vi "UI_Alarm_Settings_Sensor.vi"() -> ()   [LabVIEW 2014]
uses:
  <vilib>/addons/database/NI_Database_API.lvlib
  <vilib>/addons/database/Connection.llb/DB Tools Open Connec (String).vi
  <vilib>/addons/database/Connection.llb/Conn Execute.vi
  <vilib>/addons/database/Recordset.llb/Rec Destroy - Connection.vi
panel:
  in  "退出":bool
  in  "转速":u16(ring) items=["L0", "L1", "L2", "L3"]
  in  "径向位移":u16(ring) items=["L0", "L1", "L2", "L3"]
  in  "2X/2Y位移":u16(ring) items=["L0", "L1", "L2", "L3"]
  in  "主轴检测单元":string[][](table)
  in  "保存":bool
  in  "编辑":bool
  in  "轴向油缸力":u16(ring) items=["L0", "L1", "L2", "L3"]
  in  "径向油缸力":u16(ring) items=["L0", "L1", "L2", "L3"]
  in  "轴承外圈温度":u16(ring) items=["L0", "L1", "L2", "L3"]
  in  "声发射频率":u16(ring) items=["L0", "L1", "L2", "L3"]
  in  "声发射幅度":u16(ring) items=["L0", "L1", "L2", "L3"]
  in  "出油温度":u16(ring) items=["L0", "L1", "L2", "L3"]
  in  "摩擦力矩1":u16(ring) items=["L0", "L1", "L2", "L3"]
  in  "摩擦力矩2":u16(ring) items=["L0", "L1", "L2", "L3"]
  in  "外壳振动":u16(ring) items=["L0", "L1", "L2", "L3"]
  in  "陪试温度":u16(ring) items=["L0", "L1", "L2", "L3"]
  in  "加载单元":string[][](table)
  in  "陪试轴承润滑单元":string[][](table)
  in  "实验轴承单元":string[][](table)
  # "工作参数报警门限设置"
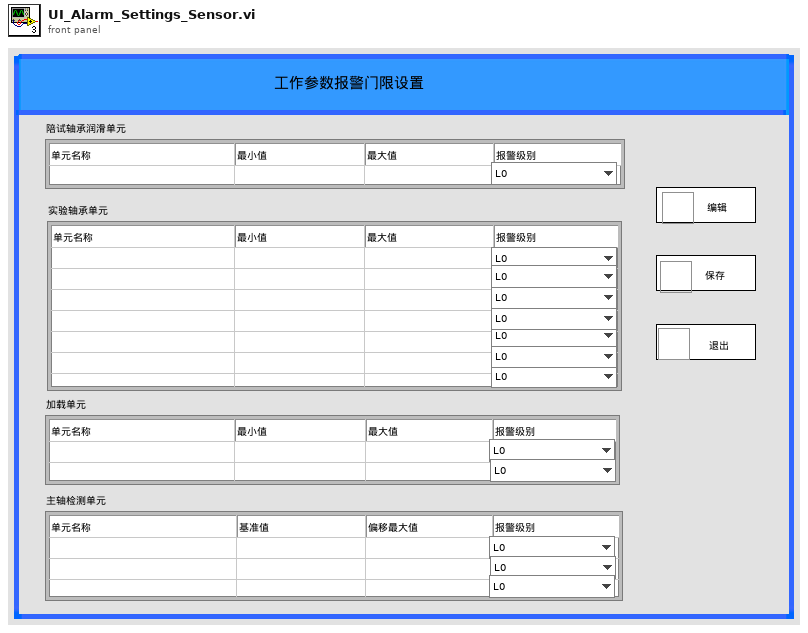
[diagram p1: front panel]
types:
  T1 = typedef "NI_Database_API.lvlib/Conn ObjectReference.ctl" = refnum<k1>
  T2 = typedef "NI_Database_API.lvlib/Rec ObjectReference.ctl" = refnum<k1>
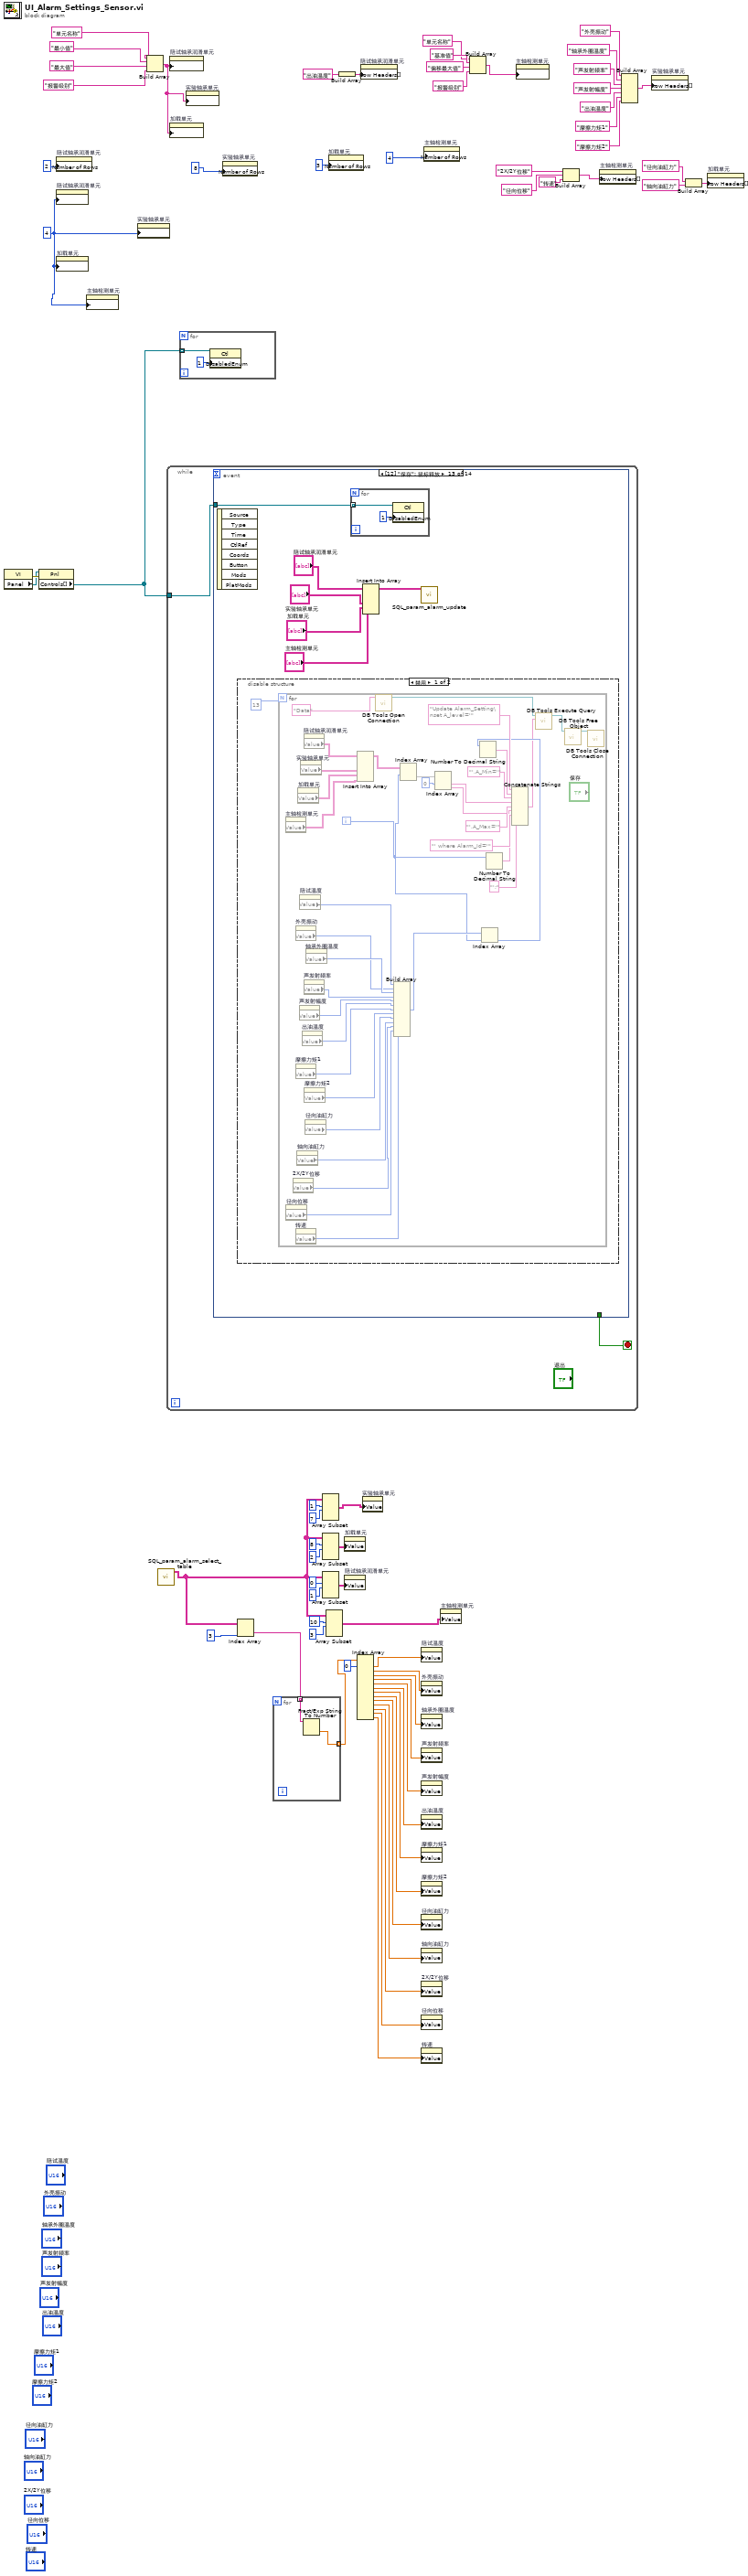
[diagram p0: block diagram]
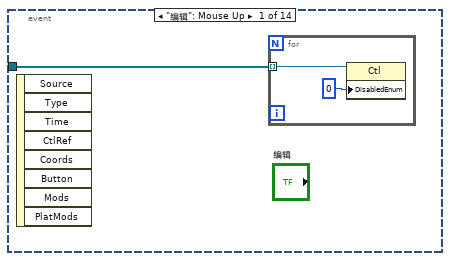
[diagram p2: hidden frame]
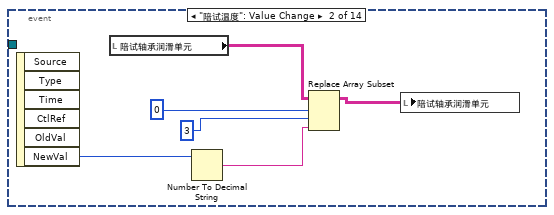
[diagram p3: hidden frame]
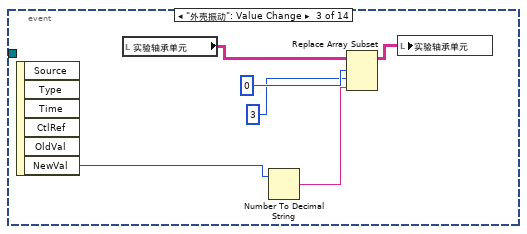
[diagram p4: hidden frame]
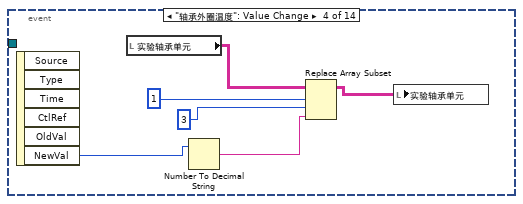
[diagram p5: hidden frame]
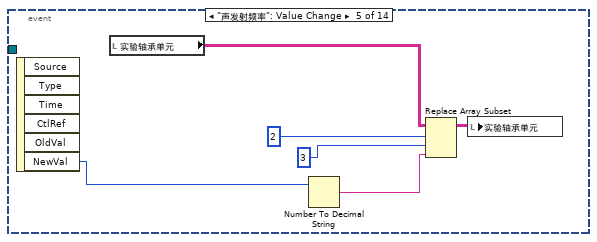
[diagram p6: hidden frame]
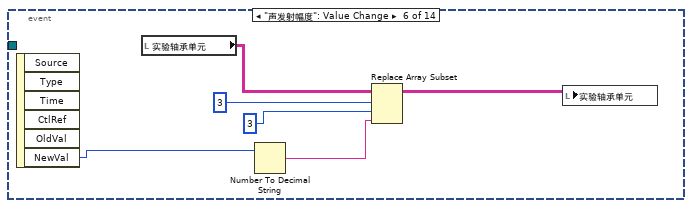
[diagram p7: hidden frame]
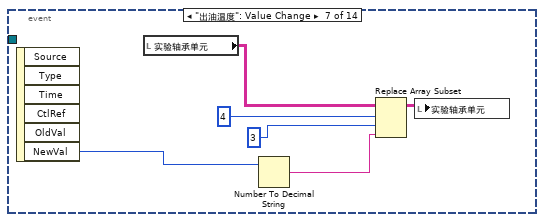
[diagram p8: hidden frame]
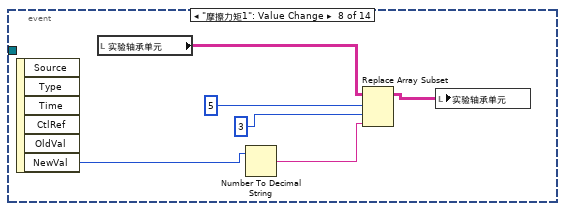
[diagram p9: hidden frame]
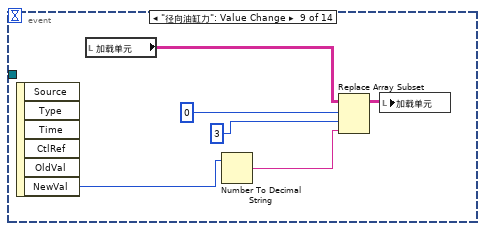
[diagram p10: hidden frame]
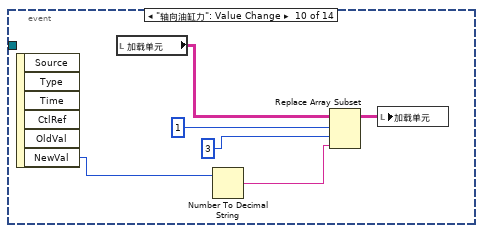
[diagram p11: hidden frame]
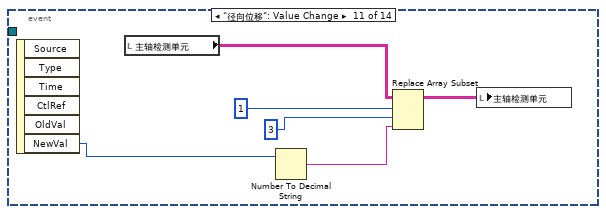
[diagram p12: hidden frame]
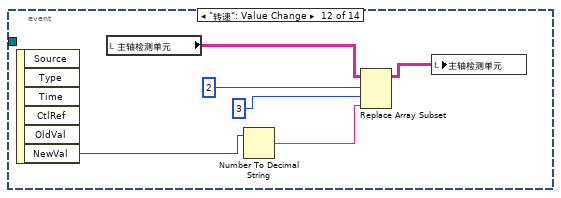
[diagram p13: hidden frame]
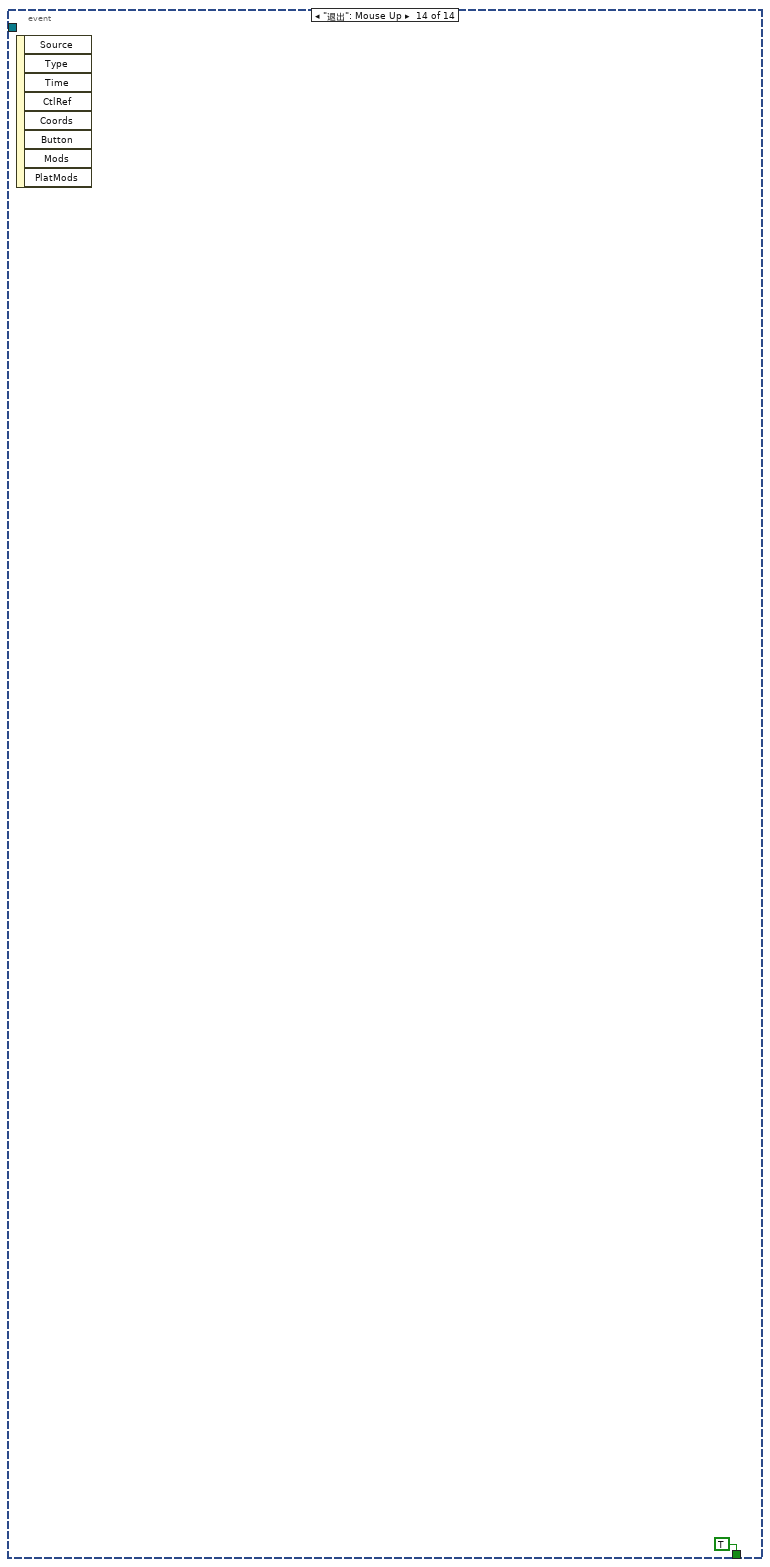
[diagram p15: hidden frame]
diagram:
  w34 = 4
  n1 = property class="VI"() -> (error out=w49:errorcluster, "Panel"=w48:refnum<vi>)  [unwired: 2 in, 1 out]
  n2 = property class="Pnl"(reference=w48, error in=w49) -> ("Controls[]"=w47:refnum<vi>[])  [unwired: 2 out]
  n3 = property on="陪试轴承润滑单元" class="Tbl (严格)"("Number of Rows"=2) -> ()  [unwired: 2 in, 2 out]
  n4 = property on="陪试轴承润滑单元" class="Tbl (严格)"("Number of Columns"=w34) -> ()  [unwired: 2 in, 2 out]
  n5 = property on="加载单元" class="Tbl (严格)"("Number of Columns"=w34) -> ()  [unwired: 2 in, 2 out]
  n6 = property on="主轴检测单元" class="Tbl (严格)"("Number of Columns"=w34) -> ()  [unwired: 2 in, 2 out]
  n7 = property on="实验轴承单元" class="Tbl (严格)"("Number of Columns"=w34) -> ()  [unwired: 2 in, 2 out]
  n8 = Build Array("单元名称", "最小值", "最大值", "报警级别") -> (w38:string[])
  n9 = call "SQL_param_alarm_select_table.vi"() -> ("表格控件"=w4:string[][])  [unwired: 10 in, 1 out]
  n10 = while {
    tunnel: w47 -> [w67]
    stop <- w66 stop-if-true
    n11 = event shown="[12] \"保存\": 鼠标释放" {
      selector: _ -> [_ _ _ _ _ _ _ _ _ _ _ _ _ _]
      dyn-events: _ -> [_ _ _ _ _ _ _ _ _ _ _ _ _ _]
      timeout: _ -> [_ _ _ _ _ _ _ _ _ _ _ _ _ _]
      tunnel: w67 -> [w68 _ _ _ _ _ _ _ _ _ _ _ w142 _]
      tunnel: [_ _ _ _ _ _ _ _ _ _ _ _ _ TRUE] -> w66
      event "编辑": Mouse Up {
        n12 = event-data() -> ()  [unwired: 1 in, 8 out]
        n13 = for {
          tunnel: w68 -> [w70] mode=indexing
          n14 = property class="Ctl"(reference=w70, "DisabledEnum"=0) -> ()  [unwired: 1 in, 2 out]
        }
      }
      event "陪试温度": Value Change {
        n15 = event-data() -> ("NewVal"=w75:u16)  [unwired: 1 in, 5 out]
        n16 = local read "陪试轴承润滑单元"() -> (w76:string[][])
        n17 = Number To Decimal String(number=w75) -> (decimal integer string=w74:string)  [unwired: 1 in]
        n18 = Replace Array Subset(array=w76, new element=w74, index (row)=0, index (col)=3) -> (w71:string[][])
        n19 = local write "陪试轴承润滑单元"(w71) -> ()
      }
      event "外壳振动": Value Change {
        n20 = event-data() -> ("NewVal"=w78:u16)  [unwired: 1 in, 5 out]
        n21 = local read "实验轴承单元"() -> (w82:string[][])
        n22 = Number To Decimal String(number=w78) -> (decimal integer string=w79:string)  [unwired: 1 in]
        n23 = Replace Array Subset(array=w82, new element=w79, index (row)=0, index (col)=3) -> (w77:string[][])
        n24 = local write "实验轴承单元"(w77) -> ()
      }
      event "轴承外圈温度": Value Change {
        n25 = event-data() -> ("NewVal"=w85:u16)  [unwired: 1 in, 5 out]
        n26 = local read "实验轴承单元"() -> (w86:string[][])
        n27 = Number To Decimal String(number=w85) -> (decimal integer string=w88:string)  [unwired: 1 in]
        n28 = Replace Array Subset(array=w86, new element=w88, index (row)=1, index (col)=3) -> (w83:string[][])
        n29 = local write "实验轴承单元"(w83) -> ()
      }
      event "声发射频率": Value Change {
        n30 = event-data() -> ("NewVal"=w90:u16)  [unwired: 1 in, 5 out]
        n31 = local read "实验轴承单元"() -> (w92:string[][])
        n32 = Number To Decimal String(number=w90) -> (decimal integer string=w94:string)  [unwired: 1 in]
        n33 = Replace Array Subset(array=w92, new element=w94, index (row)=2, index (col)=3) -> (w89:string[][])
        n34 = local write "实验轴承单元"(w89) -> ()
      }
      event "声发射幅度": Value Change {
        n35 = event-data() -> ("NewVal"=w96:u16)  [unwired: 1 in, 5 out]
        n36 = local read "实验轴承单元"() -> (w97:string[][])
        n37 = Number To Decimal String(number=w96) -> (decimal integer string=w100:string)  [unwired: 1 in]
        n38 = Replace Array Subset(array=w97, new element=w100, index (row)=3, index (col)=3) -> (w95:string[][])
        n39 = local write "实验轴承单元"(w95) -> ()
      }
      event "出油温度": Value Change {
        n40 = event-data() -> ("NewVal"=w102:u16)  [unwired: 1 in, 5 out]
        n41 = local read "实验轴承单元"() -> (w103:string[][])
        n42 = Number To Decimal String(number=w102) -> (decimal integer string=w106:string)  [unwired: 1 in]
        n43 = Replace Array Subset(array=w103, new element=w106, index (row)=4, index (col)=3) -> (w101:string[][])
        n44 = local write "实验轴承单元"(w101) -> ()
      }
      event "摩擦力矩1": Value Change {
        n45 = event-data() -> ("NewVal"=w108:u16)  [unwired: 1 in, 5 out]
        n46 = local read "实验轴承单元"() -> (w109:string[][])
        n47 = Number To Decimal String(number=w108) -> (decimal integer string=w112:string)  [unwired: 1 in]
        n48 = Replace Array Subset(array=w109, new element=w112, index (row)=5, index (col)=3) -> (w107:string[][])
        n49 = local write "实验轴承单元"(w107) -> ()
      }
      event "径向油缸力": Value Change {
        n50 = event-data() -> ("NewVal"=w114:u16)  [unwired: 1 in, 5 out]
        n51 = local read "加载单元"() -> (w115:string[][])
        n52 = Number To Decimal String(number=w114) -> (decimal integer string=w118:string)  [unwired: 1 in]
        n53 = Replace Array Subset(array=w115, new element=w118, index (row)=0, index (col)=3) -> (w113:string[][])
        n54 = local write "加载单元"(w113) -> ()
      }
      event "轴向油缸力": Value Change {
        n55 = event-data() -> ("NewVal"=w120:u16)  [unwired: 1 in, 5 out]
        n56 = local read "加载单元"() -> (w121:string[][])
        n57 = Number To Decimal String(number=w120) -> (decimal integer string=w124:string)  [unwired: 1 in]
        n58 = Replace Array Subset(array=w121, new element=w124, index (row)=1, index (col)=3) -> (w119:string[][])
        n59 = local write "加载单元"(w119) -> ()
      }
      event "径向位移": Value Change {
        n60 = event-data() -> ("NewVal"=w126:u16)  [unwired: 1 in, 5 out]
        n61 = local read "主轴检测单元"() -> (w127:string[][])
        n62 = Number To Decimal String(number=w126) -> (decimal integer string=w130:string)  [unwired: 1 in]
        n63 = Replace Array Subset(array=w127, new element=w130, index (row)=1, index (col)=3) -> (w125:string[][])
        n64 = local write "主轴检测单元"(w125) -> ()
      }
      event "转速": Value Change {
        n65 = event-data() -> ("NewVal"=w132:u16)  [unwired: 1 in, 5 out]
        n66 = local read "主轴检测单元"() -> (w133:string[][])
        n67 = Number To Decimal String(number=w132) -> (decimal integer string=w136:string)  [unwired: 1 in]
        n68 = Replace Array Subset(array=w133, new element=w136, index (row)=2, index (col)=3) -> (w131:string[][])
        n69 = local write "主轴检测单元"(w131) -> ()
      }
      event "保存": Mouse Up {
        n70 = event-data() -> ()  [unwired: 1 in, 8 out]
        n71 = disable-structure shown="禁用" {
          frame Disabled {
            n72 = for {
              N: 13 -> [_]
              i -> [w145]
              n73 = property on="主轴检测单元" class="Tbl (严格)"() -> ("Value"=w144:string[][])  [unwired: 2 in, 2 out]
              n74 = property on="径向位移" class="Ring (严格)"() -> ("Value"=w157:u16)  [unwired: 2 in, 2 out]
              n75 = property on="2X/2Y位移" class="Ring (严格)"() -> ("Value"=w156:u16)  [unwired: 2 in, 2 out]
              n76 = property on="外壳振动" class="Ring (严格)"() -> ("Value"=w147:u16)  [unwired: 2 in, 2 out]
              n77 = property on="摩擦力矩1" class="Ring (严格)"() -> ("Value"=w152:u16)  [unwired: 2 in, 2 out]
              n78 = property on="转速" class="Ring (严格)"() -> ("Value"=w158:u16)  [unwired: 2 in, 2 out]
              n79 = property on="轴向油缸力" class="Ring (严格)"() -> ("Value"=w155:u16)  [unwired: 2 in, 2 out]
              n80 = property on="加载单元" class="Tbl (严格)"() -> ("Value"=w161:string[][])  [unwired: 2 in, 2 out]
              n81 = property on="声发射幅度" class="Ring (严格)"() -> ("Value"=w150:u16)  [unwired: 2 in, 2 out]
              n82 = property on="陪试温度" class="Ring (严格)"() -> ("Value"=w159:u16)  [unwired: 2 in, 2 out]
              n83 = property on="实验轴承单元" class="Tbl (严格)"() -> ("Value"=w162:string[][])  [unwired: 2 in, 2 out]
              n84 = property on="出油温度" class="Ring (严格)"() -> ("Value"=w151:u16)  [unwired: 2 in, 2 out]
              n85 = property on="陪试轴承润滑单元" class="Tbl (严格)"() -> ("Value"=w163:string[][])  [unwired: 2 in, 2 out]
              n86 = property on="声发射频率" class="Ring (严格)"() -> ("Value"=w149:u16)  [unwired: 2 in, 2 out]
              n87 = property on="摩擦力矩2" class="Ring (严格)"() -> ("Value"=w153:u16)  [unwired: 2 in, 2 out]
              n88 = property on="径向油缸力" class="Ring (严格)"() -> ("Value"=w154:u16)  [unwired: 2 in, 2 out]
              n89 = property on="轴承外圈温度" class="Ring (严格)"() -> ("Value"=w148:u16)  [unwired: 2 in, 2 out]
              n90 = Insert Into Array(array=w163, new element #1=w162, new element #2=w161, new element #3=w144) -> (w160:string[][])  [unwired: 2 in]
              n91 = call-poly <vilib>:"DB Tools Open Connection.vi"("connection information"="Data") -> ("connection reference"=w164:T1)  [unwired: 7 in, 1 out]
              n92 = Build Array(w159, w147, w148, w149, w150, w151, w152, w153, w154, w155, w156, w157, w158) -> (w146:u16[])
              n93 = Index Array(array=w160, index (row)=w145) -> (element=w179:string[])  [unwired: 1 in]
              n94 = Index Array(array=w179, index #1=0) -> (element #1=w172:string, element #2=w173:string)  [unwired: 1 in]
              n95 = Index Array(array=w146, index=w145) -> (element=w171:u16)
              n96 = Number To Decimal String(number=w171) -> (decimal integer string=w177:string)  [unwired: 1 in]
              n97 = Number To Decimal String(number=w145) -> (decimal integer string=w167:string)  [unwired: 1 in]
              n98 = Concatenate Strings("Update Alarm_Setting\nset A_level='", w177, "',A_Min='", w172, "',A_Max='", w173, "' where Alarm_Id='", w167, "';") -> (w170:string)
              n99 = call-poly <vilib>:"DB Tools Execute Query.vi"("SQL query"=w170, "connection reference"=w164) -> ("recordset reference"=w169:T2)  [unwired: 6 in, 1 out]
              n100 = call-poly <vilib>:"DB Tools Free Object.vi"("recordset reference"=w169) -> ("connection reference"=w168:T1)  [unwired: 9 in, 1 out]
              n101 = call <vilib>:"DB Tools Close Connection.vi"("connection reference"=w168) -> ()  [unwired: 6 in, 1 out]
            }
          }
          frame Enabled {
          }
        }
        n102 = for {
          tunnel: w142 -> [w181] mode=indexing
          n103 = property class="Ctl"(reference=w181, "DisabledEnum"=1) -> ()  [unwired: 1 in, 2 out]
        }
        n104 = Insert Into Array(array="陪试轴承润滑单元", new element #1="实验轴承单元", new element #2="加载单元", new element #3="主轴检测单元") -> (w137:string[][])  [unwired: 2 in]
        n105 = call "SQL_param_alarm_update.vi"("表格控件"=w137) -> ()  [unwired: 10 in, 1 out]
      }
      event "退出": Mouse Up {
        n106 = event-data() -> ()  [unwired: 1 in, 8 out]
      }
    }
  }
  n107 = property on="陪试轴承润滑单元" class="Tbl (严格)"("Column Headers[]"=w38) -> ()  [unwired: 2 in, 2 out]
  n108 = property on="加载单元" class="Tbl (严格)"("Column Headers[]"=w38) -> ()  [unwired: 2 in, 2 out]
  n109 = for {
    tunnel: w47 -> [w184] mode=indexing
    n110 = property class="Ctl"(reference=w184, "DisabledEnum"=1) -> ()  [unwired: 1 in, 2 out]
  }
  n111 = property on="实验轴承单元" class="Tbl (严格)"("Column Headers[]"=w38) -> ()  [unwired: 2 in, 2 out]
  n112 = property on="实验轴承单元" class="Tbl (严格)"("Number of Rows"=8) -> ()  [unwired: 2 in, 2 out]
  n113 = Index Array(array=w4, index (col)=3) -> (element=w3:string[])  [unwired: 1 in]
  n114 = for {
    tunnel: [w187] -> w2 mode=indexing
    tunnel: w3 -> [w186] mode=indexing
    n115 = Fract/Exp String To Number(string=w186) -> (number=w187:dbl)  [unwired: 3 in, 1 out]
  }
  n116 = Array Subset(array=w4, index (row)=1, length (row)=7) -> (w6:string[][])  [unwired: 2 in]
  n117 = Array Subset(array=w4, index (row)=8, length (row)=2) -> (w24:string[][])  [unwired: 2 in]
  n118 = Array Subset(array=w4, index (row)=0, length (row)=1) -> (w30:string[][])  [unwired: 2 in]
  n119 = Array Subset(array=w4, index (row)=10, length (row)=3) -> (w5:string[][])  [unwired: 2 in]
  n120 = property on="加载单元" class="Tbl (严格)"("Number of Rows"=3) -> ()  [unwired: 2 in, 2 out]
  n121 = Build Array("出油温度") -> (w64:string[])
  n122 = property on="加载单元" class="Tbl (严格)"("Value"=w24) -> ()  [unwired: 2 in, 2 out]
  n123 = property on="陪试轴承润滑单元" class="Tbl (严格)"("Value"=w30) -> ()  [unwired: 2 in, 2 out]
  n124 = Index Array(array=w2, index #1=0) -> (element #1=w19:dbl, element #2=w18:dbl, element #3=w17:dbl, element #4=w16:dbl, element #5=w15:dbl, element #6=w14:dbl, element #7=w13:dbl, element #8=w12:dbl, element #9=w11:dbl, element #10=w10:dbl, element #11=w9:dbl, element #12=w8:dbl, element #13=w7:dbl)  [unwired: 12 in]
  n125 = property on="陪试轴承润滑单元" class="Tbl (严格)"("Row Headers[]"=w64) -> ()  [unwired: 2 in, 2 out]
  n126 = property on="实验轴承单元" class="Tbl (严格)"("Value"=w6) -> ()  [unwired: 2 in, 2 out]
  n127 = property on="陪试温度" class="Ring (严格)"("Value"=w19) -> ()  [unwired: 2 in, 2 out]
  n128 = property on="外壳振动" class="Ring (严格)"("Value"=w18) -> ()  [unwired: 2 in, 2 out]
  n129 = property on="轴承外圈温度" class="Ring (严格)"("Value"=w17) -> ()  [unwired: 2 in, 2 out]
  n130 = property on="声发射频率" class="Ring (严格)"("Value"=w16) -> ()  [unwired: 2 in, 2 out]
  n131 = property on="声发射幅度" class="Ring (严格)"("Value"=w15) -> ()  [unwired: 2 in, 2 out]
  n132 = property on="出油温度" class="Ring (严格)"("Value"=w14) -> ()  [unwired: 2 in, 2 out]
  n133 = property on="摩擦力矩1" class="Ring (严格)"("Value"=w13) -> ()  [unwired: 2 in, 2 out]
  n134 = property on="摩擦力矩2" class="Ring (严格)"("Value"=w12) -> ()  [unwired: 2 in, 2 out]
  n135 = property on="径向油缸力" class="Ring (严格)"("Value"=w11) -> ()  [unwired: 2 in, 2 out]
  n136 = property on="轴向油缸力" class="Ring (严格)"("Value"=w10) -> ()  [unwired: 2 in, 2 out]
  n137 = property on="2X/2Y位移" class="Ring (严格)"("Value"=w9) -> ()  [unwired: 2 in, 2 out]
  n138 = property on="径向位移" class="Ring (严格)"("Value"=w8) -> ()  [unwired: 2 in, 2 out]
  n139 = property on="转速" class="Ring (严格)"("Value"=w7) -> ()  [unwired: 2 in, 2 out]
  n140 = property on="主轴检测单元" class="Tbl (严格)"("Number of Rows"=4) -> ()  [unwired: 2 in, 2 out]
  n141 = property on="主轴检测单元" class="Tbl (严格)"("Value"=w5) -> ()  [unwired: 2 in, 2 out]
  n142 = Build Array("单元名称", "基准值", "偏移最大值", "报警级别") -> (w33:string[])
  n143 = property on="主轴检测单元" class="Tbl (严格)"("Column Headers[]"=w33) -> ()  [unwired: 2 in, 2 out]
  n144 = Build Array("2X/2Y位移", "径向位移", "转速") -> (w35:string[])
  n145 = property on="主轴检测单元" class="Tbl (严格)"("Row Headers[]"=w35) -> ()  [unwired: 2 in, 2 out]
  n146 = Build Array("外壳振动", "轴承外圈温度", "声发射频率", "声发射幅度", "出油温度", "摩擦力矩1", "摩擦力矩2") -> (w39:string[])
  n147 = property on="实验轴承单元" class="Tbl (严格)"("Row Headers[]"=w39) -> ()  [unwired: 2 in, 2 out]
  n148 = Build Array("径向油缸力", "轴向油缸力") -> (w58:string[])
  n149 = property on="加载单元" class="Tbl (严格)"("Row Headers[]"=w58) -> ()  [unwired: 2 in, 2 out]
